vi "Setm DEC wrapper.vi"(7 "bAckEna":i32, 8 "error in (no error)":errorcluster caption="错误输入（无错误）", 9 "iValue":i32, 10 "dwCanNodeId":u32, 11 "dwDevIndex":u32) -> (0 "error out":errorcluster caption="错误输出", 3 "function return":u32, 4 "pRtnValue out":i32)   [LabVIEW 2016, in "UISimCanFunc_wrapper.lvlib"]
doc: "_declspec (dllexport) DWORD SetmDEC_wrapper(DWORD dwDevIndex, DWORD dwCanNodeId, INT iValue, BOOL bAckEna, PINT pRtnValue);"
uses:
  <userlib>/UISimCanFunc_wrapper/UISimCanFunc_wrapper.lvlib
  <userlib>/UISimCanFunc_wrapper/UISimCanFunc_wrapper.dll
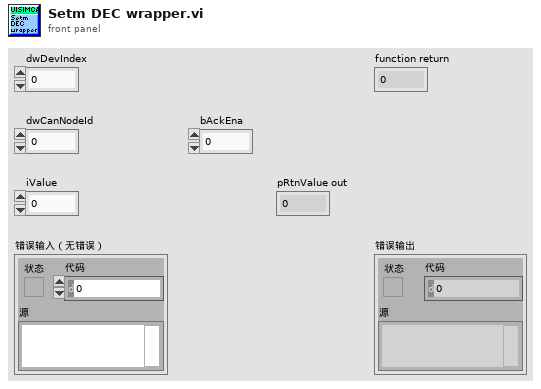
[diagram p1: front panel]
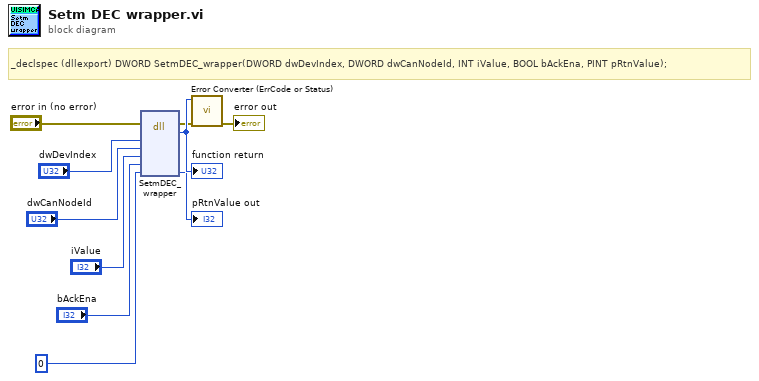
[diagram p0: block diagram]
diagram:
  # "_declspec (dllexport) DWORD SetmDEC_wrapper(DWORD dwDevIndex, DWORD dwCanNodeId, INT iValue, BOOL bAckEna, PINT pRtnValue);"
  n1 = dll-call lib="C:/Program Files (x86)/National Instruments/LabVIEW 2016/user.lib/UISimCanFunc_wrapper/UISimCanFunc_wrapper.*" fn="SetmDEC_wrapper"(error in="error in (no error)", "dwDevIndex"="dwDevIndex", "dwCanNodeId"="dwCanNodeId", "iValue"="iValue", "bAckEna"="bAckEna", "pRtnValue"=0) -> (error out=w2:errorcluster, w10:u32, "pRtnValue"=→"pRtnValue out":i32)  [unwired: 6 in, 1 out]
  "function return" <- w10
  n2 = call <userlib>:"Error Converter (ErrCode or Status).vi"("error in (no error)"=w2, "error code"=w10) -> ("error out"=→"error out":errorcluster)  [unwired: 9 in]
